vi "HFRR ADV v02.vi"() -> ()   [LabVIEW 2025] (continued)
            n2938 = property on="Sample Temperature ( °C )" class="XYGraph (strict)"("X Scale.Range:Minimum"=0.0, "X Scale.Range:Maximum"=75.0, "Y Scale.Range:Minimum"=58.0, "Y Scale.Range:Maximum"=62.0) -> ()  [unwired: 2 in, 2 out]
          }
        }
        n2939 = case shown="True" "RSTV1 3" {
          frame False {
          }
          frame True {
            n2940 = property on="Air Temperature  ( °C )" class="XYGraph (strict)"("Y Scale.Display Format:Precision"=u8 2 ("Y Scale.Format & Precision:Precision")) -> ()  [unwired: 2 in, 2 out]
            n2941 = property on="Air Temperature  ( °C )" class="XYGraph (strict)"("X Scale.Range:Minimum"=0.0 ("Y Scale.Range:Minimum"), "X Scale.Range:Maximum"=75.0 ("Y Scale.Range:Maximum"), "Y Scale.Range:Minimum"=20.0 ("X Scale.Range:Minimum"), "Y Scale.Range:Maximum"=26.0 ("X Scale.Range:Maximum")) -> ()  [unwired: 2 in, 2 out]
          }
        }
        n2942 = case shown="True" "RSTV1 4" {
          frame False {
          }
          frame True {
            n2943 = property on="Stroke ( mm )" class="XYGraph (strict)"("Y Scale.Display Format:Precision"=u8 2 ("Y Scale.Format & Precision:Precision")) -> ()  [unwired: 2 in, 2 out]
            n2944 = property on="Stroke ( mm )" class="XYGraph (strict)"("X Scale.Range:Minimum"=0.0 ("Y Scale.Range:Maximum"), "X Scale.Range:Maximum"=75.0 ("X Scale.Range:Minimum"), "Y Scale.Range:Minimum"=0.98, "Y Scale.Range:Maximum"=1.02) -> ()  [unwired: 2 in, 2 out]
          }
        }
        n2945 = case shown="True" "rstv2" {
          frame False {
          }
          frame True {
            n2946 = property on="Coefficient Of Friction" class="XYGraph (strict)"("Y Scale.Display Format:Precision"=u8 3 ("Y Scale.Format & Precision:Precision")) -> ()  [unwired: 2 in, 2 out]
            n2947 = property on="Coefficient Of Friction" class="XYGraph (strict)"("X Scale.Range:Minimum"=0.0 ("Y Scale.Range:Maximum"), "X Scale.Range:Maximum"=75.0, "Y Scale.Range:Minimum"=0.0, "Y Scale.Range:Maximum"=1.0 ("X Scale.Range:Minimum")) -> ()  [unwired: 2 in, 2 out]
          }
        }
        n2948 = case shown="True" "RST CP 3" {
          frame False {
          }
          frame True {
            n2949 = property on="Air Temp ( °C ) vs Humidity ( % RH )" class="XYGraph (strict)"("X Scale.Range:Minimum"=18.0, "X Scale.Range:Maximum"=28.0 ("X Scale.Range:Minimum"), "Y Scale.Range:Minimum"=30.0 ("X Scale.Range:Minimum"), "Y Scale.Range:Maximum"=70.0 ("X Scale.Range:Minimum")) -> ()  [unwired: 2 in, 2 out]
          }
        }
        n2950 = case shown="True" "OPEN 1" {
          frame False {
          }
          frame True {
            (unwired) 0  # existing file
            w3705 = "Choose a datalog file to open"  # prompt
            n2951 = local write "OPEN 1"(FALSE ("OPEN 1")) -> ()
            n2952 = String To Path(string="C:\\LAB-IQ\\Data\\") -> (path=w3690:path)
            n2953 = File Dialog(6:"*.dgf" ("pattern"), 7:w3705, 11:w3690) -> (0:w3688:errorcluster, 3:w3696:path)  [unwired: 4 in, 2 out]
            n2954 = Unbundle(w3688) -> ()  [unwired: 3 out]
            n2955 = Strip Path(path=w3696) -> (name=w3695:string)  [unwired: 1 out]
            n2956 = Path To String(path=w3696) -> (string=w3691:string)
            "string1" <- w3691
            n2957 = Match Pattern(string=w3695, regular expression=".dgf") -> (before substring=→"String Control":string)  [unwired: 1 in, 3 out]
            n2958 = Match Pattern(string=w3691, regular expression=".dgf" ("substring (\"\")")) -> (before substring=w3701:string)  [unwired: 1 in, 3 out]
            n2959 = Concatenate Strings(w3701, ".duf" ("Substring")) -> (w3697:string)
            n2960 = String To Path(string=w3697) -> (path=w3702:path)
            n2961 = call <vilib>:"Read Characters From File.vi"("file path (dialog if empty)"=w3702, "start of read offset (chars.:0)"=60 ("start of read offset (chars.: 0)")) -> ("character string"=→"String Control 2":string)  [unwired: 4 in, 3 out]
          }
        }
        n2962 = case shown="True" "OPEN 2" {
          frame False {
          }
          frame True {
            (unwired) 0  # existing file
            w3723 = "Choose a datalog file to open"  # prompt
            n2963 = local write "OPEN 2"(FALSE ("OPEN 1")) -> ()
            n2964 = String To Path(string="C:\\LAB-IQ\\Data\\") -> (path=w3708:path)
            n2965 = File Dialog(6:"*.dgf" ("pattern"), 7:w3723, 11:w3708) -> (0:w3706:errorcluster, 3:w3714:path)  [unwired: 4 in, 2 out]
            n2966 = Unbundle(w3706) -> ()  [unwired: 3 out]
            n2967 = Strip Path(path=w3714) -> (name=w3712:string)  [unwired: 1 out]
            n2968 = Path To String(path=w3714) -> (string=w3709:string)
            "string1 2" <- w3709
            n2969 = Match Pattern(string=w3712, regular expression=".dgf") -> (before substring=→"String Control 3":string)  [unwired: 1 in, 3 out]
            n2970 = Match Pattern(string=w3709, regular expression=".dgf" ("substring (\"\")")) -> (before substring=w3720:string)  [unwired: 1 in, 3 out]
            n2971 = Concatenate Strings(w3720, ".duf" ("Substring")) -> (w3717:string)
            n2972 = String To Path(string=w3717) -> (path=w3715:path)
            n2973 = call <vilib>:"Read Characters From File.vi"("file path (dialog if empty)"=w3715, "start of read offset (chars.:0)"=60 ("start of read offset (chars.: 0)")) -> ("character string"=→"String Control 4":string)  [unwired: 4 in, 3 out]
          }
        }
        n2974 = case shown="True" "OPEN 3" {
          frame False {
          }
          frame True {
            (unwired) 0  # existing file
            w3741 = "Choose a datalog file to open"  # prompt
            n2975 = local write "OPEN 3"(FALSE ("OPEN 1")) -> ()
            n2976 = String To Path(string="C:\\LAB-IQ\\Data\\") -> (path=w3726:path)
            n2977 = File Dialog(6:"*.dgf" ("pattern"), 7:w3741, 11:w3726) -> (0:w3724:errorcluster, 3:w3732:path)  [unwired: 4 in, 2 out]
            n2978 = Unbundle(w3724) -> ()  [unwired: 3 out]
            n2979 = Strip Path(path=w3732) -> (name=w3730:string)  [unwired: 1 out]
            n2980 = Path To String(path=w3732) -> (string=w3727:string)
            "string1 3" <- w3727
            n2981 = Match Pattern(string=w3730, regular expression=".dgf") -> (before substring=→"String Control 5":string)  [unwired: 1 in, 3 out]
            n2982 = Match Pattern(string=w3727, regular expression=".dgf" ("substring (\"\")")) -> (before substring=w3737:string)  [unwired: 1 in, 3 out]
            n2983 = Concatenate Strings(w3737, ".duf" ("Substring")) -> (w3734:string)
            n2984 = String To Path(string=w3734) -> (path=w3738:path)
            n2985 = call <vilib>:"Read Characters From File.vi"("file path (dialog if empty)"=w3738, "start of read offset (chars.:0)"=60 ("start of read offset (chars.: 0)")) -> ("character string"=→"String Control 6":string)  [unwired: 4 in, 3 out]
          }
        }
        n2986 = case shown="True" "OPEN 4" {
          frame False {
          }
          frame True {
            (unwired) 0  # existing file
            w3759 = "Choose a datalog file to open"  # prompt
            n2987 = local write "OPEN 4"(FALSE ("OPEN 1")) -> ()
            n2988 = String To Path(string="C:\\LAB-IQ\\Data\\") -> (path=w3744:path)
            n2989 = File Dialog(6:"*.dgf" ("pattern"), 7:w3759, 11:w3744) -> (0:w3742:errorcluster, 3:w3750:path)  [unwired: 4 in, 2 out]
            n2990 = Unbundle(w3742) -> ()  [unwired: 3 out]
            n2991 = Strip Path(path=w3750) -> (name=w3748:string)  [unwired: 1 out]
            n2992 = Path To String(path=w3750) -> (string=w3745:string)
            "string1 4" <- w3745
            n2993 = Match Pattern(string=w3748, regular expression=".dgf") -> (before substring=→"String Control 7":string)  [unwired: 1 in, 3 out]
            n2994 = Match Pattern(string=w3745, regular expression=".dgf" ("substring (\"\")")) -> (before substring=w3755:string)  [unwired: 1 in, 3 out]
            n2995 = Concatenate Strings(w3755, ".duf" ("Substring")) -> (w3752:string)
            n2996 = String To Path(string=w3752) -> (path=w3756:path)
            n2997 = call <vilib>:"Read Characters From File.vi"("file path (dialog if empty)"=w3756, "start of read offset (chars.:0)"=60 ("start of read offset (chars.: 0)")) -> ("character string"=→"String Control 8":string)  [unwired: 4 in, 3 out]
          }
        }
      }
      frame "About" {
        # "Elapsed time\ncof\nstroke\nmean pos\nTemp\nHumidity"
        n2998 = disable-structure shown="Disabled" {
          frame Disabled {
            n2999 = case shown="True" "Export" {
              frame False {
              }
              frame True {
                w3781 = "                                      " ("string")
                w3783 = "\r"
                (unwired) i16 6 ("width (-)")
                w3860 = "\r"
                w3792 = "\r"
                n3000 = local write "Export"(FALSE ("Export")) -> ()
                n3001 = local read "String 29"() -> (w3829:string)
                n3002 = local read "String 34"() -> (w3817:string)
                n3003 = local read "String 35"() -> (w3812:string)
                n3004 = local read "String 37"() -> (w3808:string)
                n3005 = local read "String 36"() -> (w3805:string)
                n3006 = local read "String 38"() -> (w3802:string)
                n3007 = local read "String 39"() -> (w3799:string)
                n3008 = Match Pattern(string=w3829, regular expression=".dwm") -> (before substring=w3825:string)  [unwired: 1 in, 3 out]
                "before substring" <- w3825
                n3009 = local read "S 38"() -> (w3820:string)
                n3010 = local read "S 39"() -> (w3813:string)
                n3011 = local read "Temperature before test 2"() -> (w3849:dbl)
                n3012 = local read "Temperature after test 2"() -> (w3854:dbl)
                n3013 = local read "Humidity before test 2"() -> (w3835:dbl)
                n3014 = local read "Humidity after test 2"() -> (w3850:dbl)
                n3015 = local read "MWSD 2"() -> (w3846:dbl)
                n3016 = local read "WS1.4 2"() -> (w3862:dbl)
                n3017 = local read "HCF 2"() -> (w3858:dbl)
                n3018 = local read "AVP 2"() -> (w3847:dbl)
                n3019 = Concatenate Strings("1," ("string"), w3820) -> (w3819:string)
                n3020 = Concatenate Strings("2," ("string"), w3817) -> (w3816:string)
                n3021 = Concatenate Strings("3," ("string"), w3813) -> (w3815:string)
                n3022 = Concatenate Strings("4," ("string"), w3812) -> (w3811:string)
                n3023 = Concatenate Strings("5," ("string"), w3808) -> (w3809:string)
                n3024 = Concatenate Strings("6," ("string"), w3805) -> (w3806:string)
                n3025 = Concatenate Strings("7," ("string"), w3802) -> (w3803:string)
                n3026 = Concatenate Strings("8," ("string"), w3799) -> (w3800:string)
                n3027 = local read "Sample ID"() -> (w3867:string)
                n3028 = case shown="\"xlx\"" "Select File Type" {
                  tunnel: w3825 -> [w3870 w3872 w3874]
                  tunnel: [w3868 w3873 w3875] -> w3824
                  frame "xlx" {
                    n3029 = Concatenate Strings(w3870, ".xls" ("string")) -> (w3868:string)
                  }
                  frame "csv" {
                    n3030 = Concatenate Strings(w3872, ".csv" ("string")) -> (w3873:string)
                  }
                  frame "txt" {
                    n3031 = Concatenate Strings(w3874, ".txt" ("string")) -> (w3875:string)
                  }
                }
                n3032 = local read "Test Date"() -> (w3866:string)
                n3033 = local read "String 45"() -> (w3780:string)
                n3034 = local read "String 31"() -> (w3865:string)
                n3035 = local read "String 32"() -> (w3864:string)
                n3036 = local read "TITTLE"() -> (w3788:string)
                n3037 = Number To Fractional String(number=w3835, width (-)=i16 6, precision (6)=i16 2) -> (F-format string=w3834:string)  [unwired: 1 in]
                n3038 = Number To Fractional String(number=w3849, width (-)=i16 6, precision (6)=i16 2) -> (F-format string=w3855:string)  [unwired: 1 in]
                n3039 = Number To Fractional String(number=w3850, width (-)=i16 6, precision (6)=i16 2) -> (F-format string=w3848:string)  [unwired: 1 in]
                n3040 = Number To Fractional String(number=w3854, width (-)=i16 6, precision (6)=i16 2) -> (F-format string=w3853:string)  [unwired: 1 in]
                n3041 = Number To Fractional String(number=w3846, width (-)=i16 6, precision (6)=i16 2) -> (F-format string=w3844:string)  [unwired: 1 in]
                n3042 = Number To Fractional String(number=w3847, width (-)=i16 6, precision (6)=i16 2) -> (F-format string=w3845:string)  [unwired: 1 in]
                n3043 = Number To Fractional String(number=w3858, width (-)=i16 6, precision (6)=i16 2) -> (F-format string=w3859:string)  [unwired: 1 in]
                n3044 = Number To Fractional String(number=w3862, precision (6)=i16 2) -> (F-format string=w3863:string)  [unwired: 2 in]
                n3045 = local read "s.NO"() -> (w3782:string)
                n3046 = Concatenate Strings("=" ("string"), w3788) -> (w3787:string)
                n3047 = Concatenate Strings("S.No," ("string"), "                                       Parameters" ("string")) -> (w3793:string)
                n3048 = Concatenate Strings(w3860, w3819, w3834, w3860, w3816, w3855, w3860, w3815, w3848, w3860, w3811, w3853, w3860, w3809, w3844, w3860, w3806, w3845, w3860, w3803, w3859, w3860, w3800, w3863) -> (w3822:string)
                n3049 = Concatenate Strings(w3792, "," ("string"), w3780, w3782, w3781, w3864, w3867, w3781, w3865, w3866, w3792) -> (w3790:string)
                n3050 = local read "Tested by"() -> (w3796:string)
                n3051 = local read "String 33"() -> (w3797:string)
                n3052 = Concatenate Strings("," ("string"), "                                                                             " ("string")) -> (w3785:string)
                n3053 = Concatenate Strings(w3787, w3783, w3790, w3783, w3793, w3822, w3783, w3785, w3797, w3796) -> (→"export":string)
                n3054 = String To Path(string=w3824) -> (path=w3831:path)
                n3055 = local read "export"() -> (w3826:string)
                n3056 = call <vilib>:"Write Characters To File.vi"("append to file? (new file:F)"=FALSE, "character string"=w3826, "file path (dialog if empty)"=w3831) -> ()  [unwired: 2 in, 1 out]
              }
            }
          }
          frame Enabled {
          }
        }
        n3057 = case shown="True" "OK Button 17" {
          frame False {
          }
          frame True {
            (unwired) 0  # existing file
            w4084 = "Choose a datalog file to open"  # prompt
            n3058 = local write "OK Button 17"(FALSE ("OK Button 17")) -> ()
            n3059 = local read "String"() -> (w4079:string)
            n3060 = String To Path(string=w4079) -> (path=w4080:path)
            n3061 = File Dialog(6:"*.duf" ("pattern"), 7:w4084, 11:w4080) -> (0:w4071:errorcluster, 3:w4090:path)  [unwired: 4 in, 2 out]
            n3062 = Unbundle(w4071) -> ()  [unwired: 3 out]
            n3063 = Open/Create/Replace File "Open File"(file path (use dialog)=w4090) -> (refnum out=w4082:refnum<file>)  [unwired: 5 in, 2 out]
            n3064 = Strip Path(path=w4090) -> (name=w4088:string)  [unwired: 1 out]
            n3065 = Path To String(path=w4090) -> (string=w4073:string)
            n3066 = while {
              tunnel: w4082 -> [w4094]
              i -> [w4091]
              stop <- w4092 continue-if-true
              (unwired) TRUE ("line mode (F)")
              n3067 = Read from Text File "Read File"(file (use dialog)=w4094) -> (text=w4093:string)  [unwired: 3 in, 3 out]
              n3068 = local write "Numeric 16"(w4091) -> ()
              n3069 = String Length(string=w4093) -> (length=w4096:i32)
              n3070 = Greater?(x=w4096, y=1) -> (0:w4092:bool)
            }
            n3071 = local write "String 29"(w4073) -> ()
            n3072 = Search and Replace String(input string=w4073, search string=".duf", replace string=".dgf" ("replace string (\"\")")) -> (result string=→"String Indicator 4":string)  [unwired: 5 in, 3 out]
            n3073 = Match Pattern(string=w4088, regular expression=".dwm") -> (before substring=w4072:string)  [unwired: 1 in, 3 out]
            "String Indicator" <- w4072
            n3074 = Match Pattern(string=w4073, regular expression=".dwm" ("substring (\"\")")) -> (before substring=w4074:string)  [unwired: 1 in, 3 out]
            "String Indicator 3" <- w4074
            n3075 = local write "TITTLE 2"(w4072) -> ()
            n3076 = String To Path(string=w4074) -> (path=w4081:path)
            "path" <- w4081
            n3077 = call <vilib>:"Read Characters From File.vi"("file path (dialog if empty)"=w4081, "start of read offset (chars.:0)"=60 ("start of read offset (chars.: 0)")) -> ("character string"=→"String Indicator 2":string)  [unwired: 4 in, 3 out]
          }
        }
        n3078 = call <vilib>:"Query Available Printers.vi"() -> ("system configured printers"=w3773:string[])  [unwired: 9 in, 2 out]
        "System Configured Printers 2" <- w3773
        n3079 = local read "OK Button 16"() -> (w3770:bool)
        n3080 = case shown="True" "OK Button 16" {
          frame False {
          }
          frame True {
            n3081 = stacked-sequence {
              frame #0 {
                n3082 = local read "Numeric 16"() -> (w4098:i32)
                n3083 = local write "Numeric 10"(w4098) -> ()
              }
              frame #1 {
                n3084 = local read "String 29"() -> (w4101:string)
                n3085 = String To Path(string=w4101) -> (path=w4100:path)
                n3086 = Open/Create/Replace File "Open File"(file path (use dialog)=w4100) -> (refnum out=w4102:refnum<file>)  [unwired: 5 in, 2 out]
                n3087 = for {
                  N: 16 -> [_]
                  tunnel: w4102 -> [w4109]
                  i -> [w4105]
                  (unwired) TRUE ("line mode (F)")
                  n3088 = Read from Text File "Read File"(file (use dialog)=w4109) -> (text=w4103:string)  [unwired: 3 in, 3 out]
                  n3089 = Match Pattern(string=w4103, regular expression="(") -> (after substring=w4108:string)  [unwired: 1 in, 3 out]
                  n3090 = Match Pattern(string=w4108, regular expression=")") -> (before substring=w4104:string)  [unwired: 1 in, 3 out]
                  n3091 = case shown="1" w4105 {
                    tunnel: w4104 -> [w4110 w4111 _ _ w4112 w4113 w4114 w4116 w4118 w4120 w4122 w4124 w4126 w4128 _]
                    tunnel: w4103 -> [_ _ _ _ _ _ _ _ _ _ _ _ _ _ _]
                    frame 0 {
                      "TITTLE" <- w4110
                    }
                    frame 1 {
                      "Sample ID" <- w4111
                    }
                    frame 2 {
                    }
                    frame 3 {
                    }
                    frame 4 {
                      "Test Date" <- w4112
                    }
                    frame 5 {
                      "Tested by" <- w4113
                    }
                    frame 6 {
                      n3092 = Fract/Exp String To Number(string=w4114) -> (number=→"Humidity before test 2":dbl)  [unwired: 3 in, 1 out]
                    }
                    frame 7 {
                      n3093 = Fract/Exp String To Number(string=w4116) -> (number=→"Temperature before test 2":dbl)  [unwired: 3 in, 1 out]
                    }
                    frame 8 {
                      n3094 = Fract/Exp String To Number(string=w4118) -> (number=→"Humidity after test 2":dbl)  [unwired: 3 in, 1 out]
                    }
                    frame 9 {
                      n3095 = Fract/Exp String To Number(string=w4120) -> (number=→"Temperature after test 2":dbl)  [unwired: 3 in, 1 out]
                    }
                    frame 10 {
                      n3096 = Fract/Exp String To Number(string=w4122) -> (number=→"MWSD 2":dbl)  [unwired: 3 in, 1 out]
                    }
                    frame 11 {
                      n3097 = Fract/Exp String To Number(string=w4124) -> (number=→"AVP 2":dbl)  [unwired: 3 in, 1 out]
                    }
                    frame 12 {
                      n3098 = Fract/Exp String To Number(string=w4126) -> (number=→"HCF 2":dbl)  [unwired: 3 in, 1 out]
                    }
                    frame 13 {
                      n3099 = Fract/Exp String To Number(string=w4128) -> (number=→"WS1.4 2":dbl)  [unwired: 3 in, 1 out]
                    }
                    frame 14, Default {
                    }
                  }
                }
              }
              frame #2 {
              }
            }
            n3100 = local write "OK Button 16"(FALSE ("OK Button 13")) -> ()
          }
        }
        n3101 = Index Array(array=w3773, index="Select Printer 3") -> (element=w3775:string)
        "Selected Printer" <- w3775
        n3102 = case shown="True" w3770 {
          frame False {
          }
          frame True {
            n3103 = flat-sequence {
              frame #0 {
              }
              frame #1 {
                n3104 = Wait (ms)(milliseconds to wait=u32 100) -> ()  [unwired: 1 out]
              }
              frame #2 {
                n3105 = local write "OK Button 16"(FALSE ("Print 3")) -> ()
              }
            }
          }
        }
        n3106 = case shown="True" "Print" {
          tunnel: w3775 -> [_ w4067]
          frame False {
          }
          frame True {
            (unwired) i16 6 ("width (-)")
            (unwired) "TESTED BY : "
            (unwired) "TESTED DATE :"
            (unwired) "SAMPLE ID : "
            (unwired) "SAMPLE DESIGN : "
            w4025 = "\r"
            w4042 = "\r"
            # "add image"
            n3107 = local read "Sample ID"() -> (w4015:string)
            n3108 = local read "Tested by"() -> (w4018:string)
            n3109 = local read "String 34"() -> (w4005:string)
            n3110 = local read "String 45"() -> (w3985:string)
            n3111 = local read "String 35"() -> (w4000:string)
            n3112 = local read "String 37"() -> (w3998:string)
            n3113 = local read "String 32"() -> (w4020:string)
            n3114 = local read "String 36"() -> (w3995:string)
            n3115 = local read "String 31"() -> (w4019:string)
            n3116 = local read "Test Date"() -> (w4016:string)
            n3117 = local read "String 33"() -> (w4021:string)
            n3118 = local read "String 38"() -> (w3991:string)
            n3119 = local read "String 39"() -> (w3988:string)
            n3120 = local write "Print"(FALSE ("Print FF")) -> ()
            n3121 = local read "S 39"() -> (w4003:string)
            n3122 = local read "S 38"() -> (w4010:string)
            n3123 = local read "Temperature before test 2"() -> (w4041:dbl)
            n3124 = local read "Temperature after test 2"() -> (w4031:dbl)
            n3125 = local read "Humidity before test 2"() -> (w4056:dbl)
            n3126 = local read "Humidity after test 2"() -> (w4040:dbl)
            n3127 = local read "MWSD 2"() -> (w4045:dbl)
            n3128 = local read "WS1.4 2"() -> (w4023:dbl)
            n3129 = Concatenate Strings("2)" ("string"), w4005) -> (w4006:string)
            n3130 = Concatenate Strings("3)" ("string"), w4003) -> (w4004:string)
            n3131 = Concatenate Strings("1)" ("string"), w4010) -> (w4009:string)
            n3132 = Concatenate Strings("4)" ("string"), w4000) -> (w4001:string)
            n3133 = Concatenate Strings("5)" ("string"), w3998) -> (w3997:string)
            n3134 = Concatenate Strings("6)" ("string"), w3995) -> (w3994:string)
            n3135 = Concatenate Strings("7)" ("string"), w3991) -> (w3992:string)
            n3136 = Concatenate Strings("8)" ("string"), w3988) -> (w3989:string)
            n3137 = local read "HCF 2"() -> (w4027:dbl)
            n3138 = local read "AVP 2"() -> (w4044:dbl)
            n3139 = local read "s.NO"() -> (w3986:string)
            n3140 = call <vilib>:"New Report.vi"("report type"=enum16{"Standard Report", "HTML"}."Standard Report") -> ("report out"=w4065:refnum<class "NI_report.lvclass">, "error out"=w4064:errorcluster)  [unwired: 13 in]
            n3141 = local read "TITTLE"() -> (w4017:string)
            n3142 = Concatenate Strings(w4042, w3985, w3986, w4042, w4020, w4015, w4042, w4019, w4016, w4042, w4021, w4018, w4042) -> (w4035:string)
            "test by" <- w4035
            n3143 = Number To Fractional String(number=w4041, width (-)=i16 6, precision (6)=i16 2) -> (F-format string=w4030:string)  [unwired: 1 in]
            n3144 = Number To Fractional String(number=w4040, width (-)=i16 6, precision (6)=i16 2) -> (F-format string=w4043:string)  [unwired: 1 in]
            n3145 = Number To Fractional String(number=w4056, width (-)=i16 6, precision (6)=i16 2) -> (F-format string=w4061:string)  [unwired: 1 in]
            n3146 = Number To Fractional String(number=w4045, width (-)=i16 6, precision (6)=i16 2) -> (F-format string=w4047:string)  [unwired: 1 in]
            n3147 = Number To Fractional String(number=w4031, width (-)=i16 6, precision (6)=i16 2) -> (F-format string=w4032:string)  [unwired: 1 in]
            n3148 = Number To Fractional String(number=w4044, width (-)=i16 6, precision (6)=i16 2) -> (F-format string=w4046:string)  [unwired: 1 in]
            n3149 = Number To Fractional String(number=w4027, width (-)=i16 6, precision (6)=i16 2) -> (F-format string=w4026:string)  [unwired: 1 in]
            n3150 = Number To Fractional String(number=w4023, precision (6)=i16 2) -> (F-format string=w4022:string)  [unwired: 2 in]
            n3151 = call-dynamic "Set Report Header Text.vi"("report in"=w4065, "center header text"=w4017, "error in (no error)"=w4064) -> ("report out"=w4036:refnum<class "NI_report.lvclass">, "error out"=w4037:errorcluster)  [unwired: 11 in]
            n3152 = Concatenate Strings(w4025, w4009, w4061, w4025, w4006, w4030, w4025, w4004, w4043, w4025, w4001, w4032, w4025, w3997, w4047, w4025, w3994, w4046, w4025, w3992, w4026, w4025, w3989, w4022) -> (w4013:string)
            "export 2" <- w4013
            n3153 = call-poly <vilib>:"Append Report Text.vi"("report in"=w4036, "text"=w4035, "error in (no error)"=w4037) -> ("report out"=w4039:refnum<class "NI_report.lvclass">, "error out"=w4038:errorcluster)  [unwired: 9 in, 2 out]
            n3154 = local read "test by"() -> (w4012:string)
            n3155 = local read "TITTLE"() -> (w4014:string)
            n3156 = call-poly <vilib>:"Append Report Text.vi"("report in"=w4039, "error in (no error)"=w4038) -> ("report out"=w4060:refnum<class "NI_report.lvclass">, "error out"=w4058:errorcluster)  [unwired: 10 in, 2 out]
            n3157 = Concatenate Strings(w4014, w4013, w4012) -> (→"output":string)
            n3158 = call-poly <vilib>:"Append Report Text.vi"("report in"=w4060, "text"=w4013, "error in (no error)"=w4058) -> ("report out"=w4059:refnum<class "NI_report.lvclass">, "error out"=w4057:errorcluster)  [unwired: 9 in, 2 out]
            n3159 = call-dynamic "Print Report.vi"("report in"=w4059, "printer name (default)"=w4067, "error in (no error)"=w4057) -> ("report out"=w4069:refnum<class "NI_report.lvclass">, "error out"=w4070:errorcluster)  [unwired: 11 in]
            n3160 = call-dynamic "Dispose Report.vi"("report in"=w4069, "error in (no error)"=w4070) -> ()  [unwired: 13 in, 1 out]
          }
        }
        n3161 = case shown="True" "Print 2" {
          frame False {
          }
          frame True {
            n3162 = flat-sequence {
              frame #0 {
                n3163 = local read "s.NO"() -> (→"s.NO 2":string)
                n3164 = Wait (ms)(milliseconds to wait=u32 20) -> ()  [unwired: 1 out]
                n3165 = local read "Sample ID  3"() -> (→"Sample ID  6":string)
                n3166 = local read "Sample ID  4"() -> (→"Sample ID  7":string)
                n3167 = local read "Sample ID"() -> (→"Sample ID  2":string)
                n3168 = local read "Tested by"() -> (→"Tested by 2":string)
                n3169 = local read "Test Date"() -> (→"Test Date 2":string)
                n3170 = local read "Humidity after test 3"() -> (→"Humidity after test 4":dbl)
                n3171 = local read "Ref A Test Date :"() -> (→"TITTLE 4":string)
                n3172 = local read "Temperature before test 3"() -> (w3892:dbl)
                n3173 = local read "Temperature before test 3"() -> (→"Temperature after test 5":dbl)
                n3174 = local read "Temperature after test 3"() -> (→"Temperature after test 4":dbl)
                n3175 = local read "Humidity before test 3"() -> (→"Humidity before test 4":dbl)
                n3176 = local write "Temperature before test 3"(w3892) -> ()
                n3177 = local read "image data"() -> (w3883:T2)
                n3178 = String To Path(string="C:\\LAB-IQ\\im\\Temp_resized.jpg") -> (path=w3884:path)
                "path 2" <- w3884
                n3179 = call <vilib>:"Write JPEG File.vi"("image data"=w3883, "path to JPEG file"=w3884) -> ()  [unwired: 8 in, 2 out]
                "Ref A Test Date :" <- "Ref A Test Date :"
                "Ref B Test Date :" <- "Ref B Test Date :"
                "Ref B Scar Value :" <- "Ref B Scar Value :"
                "Ref A Scar Value :" <- "Ref A Scar Value :"
              }
              frame #1 {
                (unwired) HTML_Report_Image_Alignment."MIDDLE" ("alignment (default)")
                w3920 = u16 0 items=["portrait", "landscape"] ("orientation (portrait)")
                (unwired) HTML_Report_Image_Alignment."ABSMIDDLE" ("alignment (default)")
                (unwired) "TESTED BY : "
                (unwired) "TESTED DATE :"
                (unwired) "SAMPLE ID : "
                (unwired) "SAMPLE DESIGN : "
                w3953 = "\r"
                # "add image"
                n3180 = Wait (ms)(milliseconds to wait=u32 20) -> ()  [unwired: 1 out]
                n3181 = local read "Sample ID  2"() -> (w3946:string)
                n3182 = local read "Wear Scar X"() -> (w3918:dbl)
                "Length ( microns ) 2" <- w3918
                n3183 = local read "Wear Scar Y"() -> (w3917:dbl)
                "Wear Scar Y ( microns ) :" <- w3917
                n3184 = local read "Test Date 2"() -> (w3947:string)
                n3185 = local read "Tested by 2"() -> (w3948:string)
                n3186 = local read "String 46"() -> (w3944:string)
                n3187 = local read "String 48"() -> (w3950:string)
                n3188 = local read "String 47"() -> (w3949:string)
                n3189 = local read "String 49"() -> (w3951:string)
                n3190 = local read "String 10"() -> (w3904:string)
                n3191 = local read "s.NO 2"() -> (w3945:string)
                n3192 = Add(x=w3918, y=w3917) -> (x+y=w3916:dbl)
                n3193 = call <vilib>:"New Report.vi"("report type"=enum16{"Standard Report", "HTML"}."HTML") -> ("report out"=w3924:refnum<class "NI_report.lvclass">, "error out"=w3922:errorcluster)  [unwired: 13 in]
                n3194 = Concatenate Strings(w3953, w3944, w3945, w3953, w3950, w3946, w3953, w3949, w3947, w3953, w3951, w3948, w3953) -> (→"test by 2":string)
                n3195 = Concatenate Strings("C:\\LAB-IQ\\Data\\" ("string"), w3904, ".jpg" ("string")) -> ()  [unwired: 1 out]
                n3196 = Divide(x=w3916, y=2.0) -> (x/y=→"Mean Wear ( microns) :":dbl)
                n3197 = call-dynamic "Set Report Orientation.vi"("report in"=w3924, "orientation (portrait)"=w3920, "error in (no error)"=w3922) -> ("report out"=w3923:refnum<class "NI_report.lvclass">, "error out"=w3921:errorcluster)  [unwired: 11 in]
                n3198 = for {
                  N: 5 -> [_]
                  tunnel: w3923 -> [w3974]
                  tunnel: [w3973] -> w3902
                  tunnel: w3921 -> [w3972]
                  tunnel: [w3971] -> w3901
                  n3199 = call-dynamic "Set Report Tab Width.vi"("report in"=w3974, "error in (no error)"=w3972) -> ("report out"=w3973:refnum<class "NI_report.lvclass">, "error out"=w3971:errorcluster)  [unwired: 12 in]
                }
                n3200 = local read "TITTLE"() -> (w3919:string)
                n3201 = call-dynamic "Set Report Header Text.vi"("report in"=w3902, "center header text"=w3919, "error in (no error)"=w3901) -> ("report out"=w3940:refnum<class "NI_report.lvclass">, "error out"=w3939:errorcluster)  [unwired: 11 in]
                n3202 = for {
                  N: 1 -> [_]
                  tunnel: [w3978] -> w3926
                  tunnel: [w3977] -> w3925
                  tunnel: w3940 -> [w3976]
                  tunnel: w3939 -> [w3975]
                  n3203 = call-dynamic "New Report Line.vi"("report in"=w3976, "error in (no error)"=w3975) -> ("report out"=w3978:refnum<class "NI_report.lvclass">, "error out"=w3977:errorcluster)  [unwired: 12 in]
                }
                n3204 = for {
                  N: 2 -> [_]
                  tunnel: [w3970] -> w3932
                  tunnel: [w3969] -> w3931
                  tunnel: w3926 -> [w3968]
                  tunnel: w3925 -> [w3967]
                  n3205 = call-dynamic "New Report Line.vi"("report in"=w3968, "error in (no error)"=w3967) -> ("report out"=w3970:refnum<class "NI_report.lvclass">, "error out"=w3969:errorcluster)  [unwired: 12 in]
                }
                n3206 = for {
                  N: 25 -> [_]
                  tunnel: w3932 -> [w3966]
                  tunnel: w3931 -> [w3964]
                  tunnel: [w3965] -> w3935
                  tunnel: [w3963] -> w3934
                  n3207 = call-dynamic "Set Report Tab Width.vi"("report in"=w3966, "error in (no error)"=w3964) -> ("report out"=w3965:refnum<class "NI_report.lvclass">, "error out"=w3963:errorcluster)  [unwired: 12 in]
                }
                n3208 = control-ref of="Tab Control 9"() -> (w3930:refnum<vi>)
                n3209 = call-dynamic "Append Control Image to Report.vi"("report in"=w3935, "alignment (default)"=HTML_Report_Image_Alignment."ABSMIDDLE", "ctrl reference"=w3930, "error in (no error)"=w3934) -> ("report out"=w3929:refnum<class "NI_report.lvclass">, "error out"=w3928:errorcluster)  [unwired: 8 in, 2 out]
                n3210 = for {
                  N: 3 -> [_]
                  tunnel: [w3962] -> w3913
                  tunnel: [w3961] -> w3912
                  tunnel: w3929 -> [w3960]
                  tunnel: w3928 -> [w3959]
                  n3211 = call-dynamic "New Report Line.vi"("report in"=w3960, "error in (no error)"=w3959) -> ("report out"=w3962:refnum<class "NI_report.lvclass">, "error out"=w3961:errorcluster)  [unwired: 12 in]
                }
                n3212 = for {
                  N: 100 -> [_]
                  tunnel: w3913 -> [w3958]
                  tunnel: w3912 -> [w3956]
                  tunnel: [w3957] -> w3909
                  tunnel: [w3955] -> w3907
                  n3213 = call-dynamic "Set Report Tab Width.vi"("report in"=w3958, "error in (no error)"=w3956) -> ("report out"=w3957:refnum<class "NI_report.lvclass">, "error out"=w3955:errorcluster)  [unwired: 12 in]
                }
                n3214 = String To Path(string="C:\\LAB-IQ\\im\\Temp_resized.jpg") -> (path=w3899:path)
                n3215 = call-poly <vilib>:"Append Image to Report.vi"("report in"=w3909, "path or URL of image"=w3899, "error in (no error)"=w3907) -> ("report out"=w3908:refnum<class "NI_report.lvclass">, "error out"=w3906:errorcluster)  [unwired: 9 in, 2 out]
                n3216 = call-poly <vilib>:"Open HTML Report in Browser.vi"("report in"=w3908, "error in (no error)"=w3906) -> ("report out"=w3943:refnum<class "NI_report.lvclass">, "error out"=w3942:errorcluster)  [unwired: 11 in, 1 out]
                n3217 = call-dynamic "Dispose Report.vi"("report in"=w3943, "error in (no error)"=w3942) -> ()  [unwired: 13 in, 1 out]
              }
              frame #2 {
              }
              frame #3 {
                n3218 = disable-structure shown="Disabled" {
                  frame Disabled {
                    n3219 = local read "String 10"() -> (w3983:string)
                    n3220 = Concatenate Strings("C:\\LAB-IQ-NXT\\Data\\" ("string"), w3983, ".jpg" ("string")) -> (w3981:string)
                    n3221 = String To Path(string=w3981) -> (path=w3980:path)
                    n3222 = Delete(path (use dialog)=w3980) -> ()  [unwired: 4 in, 3 out]
                  }
                  frame Enabled {
                  }
                }
                n3223 = local write "Print 2"(FALSE ("Print")) -> ()
              }
            }
          }
        }
      }
    }
    n3224 = Wait (ms)(milliseconds to wait=u32 50) -> ()  [unwired: 1 out]
    n3225 = Wait (ms)(milliseconds to wait=u32 50) -> ()  [unwired: 1 out]
    n3226 = local read "Quit"() -> (w2344:bool)
  }
  n3227 = VISA Close(VISA resource name=w46, error in (no error)=w45) -> ()  [unwired: 1 out]
  n3228 = while {
    stop <- w4134 stop-if-true
    # "DEMO"
    n3229 = local read "Auto Start Test"() -> (w4132:bool)
    n3230 = Wait (ms)(milliseconds to wait=u32 1000) -> ()  [unwired: 1 out]
    n3231 = local read "RUN"() -> (w4131:bool)
    n3232 = Or(x=w4131, y=w4132) -> (x .or. y?=w4130:bool)
    n3233 = case shown="True" w4130 {
      frame False {
      }
      frame True {
        n3234 = local read "LVDT STROKE Actual"() -> (w4136:dbl)
        n3235 = local read "DEMO MODE"() -> (w4135:bool)
        n3236 = case shown="True" w4135 {
          frame False {
          }
          frame True {
            n3237 = call-poly <vilib>:"Random Number (Range).vi"("lower bound (0)"=22.0 ("upper bound (100)"), "upper bound (100)"=24.0) -> ("number"=w4144:dbl)  [unwired: 9 in]
            n3238 = local write "AIR TEMP"(w4144) -> ()
          }
        }
        n3239 = In Range and Coerce(upper limit=1.2, x=w4136, lower limit=0.6) -> (In Range?=w4139:bool)  [unwired: 1 out]
        n3240 = call-poly <vilib>:"Random Number (Range).vi"("lower bound (0)"=0.998 ("upper bound (100)"), "upper bound (100)"=1.003) -> ("number"=w4137:dbl)  [unwired: 9 in]
        n3241 = case shown="True" w4139 {
          tunnel: [w4147 w4148] -> w4138
          tunnel: w4137 -> [_ w4148]
          tunnel: w4136 -> [w4147 _]
          frame False {
          }
          frame True {
          }
        }
        "LVDT STROKE DISPLAY" <- w4138
      }
    }
    n3242 = local read "Quit"() -> (w4134:bool)
  }
  n3243 = while {
    tunnel: [w4165] -> w52
    shift-right: [w4158] -> _
    shift-left: 0.0 -> [w4161]
    shift-right: [w4157] -> _
    shift-left: 0.0 -> [w4160]
    shift-right: [w4156] -> _
    shift-left: 100.0 ("vc_cmd") -> [w4159]
    stop <- w4165 stop-if-true
    # "PID LOGIC"
    n3244 = local read "run test Calibration"() -> (w4153:bool)
    n3245 = local read "RUN"() -> (w4163:bool)
    n3246 = local read "Auto Start Temp"() -> (w4154:bool)
    n3247 = local read "Auto Start Test"() -> (w4162:bool)
    n3248 = local read "START TEMP"() -> (w4152:bool)
    n3249 = And(x=w4154, y=w4162) -> (x .and. y?=w4155:bool)
    n3250 = Or(x=w4163, y=w4155) -> (x .or. y?=w4164:bool)
    n3251 = And(x=w4164, y=w4152) -> (x .and. y?=w4151:bool)
    n3252 = And(x=w4153, y=w4152) -> (x .and. y?=w4150:bool)
    n3253 = Or(x=w4150, y=w4151) -> (x .or. y?=w4149:bool)
    n3254 = Wait (ms)(milliseconds to wait="milliseconds to wait") -> ()  [unwired: 1 out]
    n3255 = case shown="True" w4149 {
      tunnel: [400.0 ("out_vc_cmd") w4184] -> w4156
      tunnel: [w4168 w4186] -> w4157
      tunnel: [w4168 w4185] -> w4158
      tunnel: w4161 -> [_ w4175]
      tunnel: w4160 -> [_ w4174]
      tunnel: w4159 -> [_ w4173]
      tunnel: w4153 -> [_ w4169]
      frame False {
        w4168 = 0.0 ("error_out")
      }
      frame True {
        n3256 = case shown="True" w4169 {
          tunnel: [w4193 1.0] -> w4171
          frame False {
            n3257 = local read "Set Strk"() -> (w4192:dbl)
            n3258 = Add(x=w4192, y="Add up Stroke") -> (x+y=w4193:dbl)
          }
          frame True {
          }
        }
        n3259 = local read "LVDT STROKE"() -> (w4170:dbl)
        n3260 = formula code="// Zero-Hardcode Explicit Positional-Form PID Engine\n// Inputs: target_stroke, measured_stroke, dt, prev_error, integral_accumulator_in, prev_vc_cmd\n//         kp, ki, kd, max_step_change, max_amplitude, min_amplitude, startup_cmd\n// Outputs: vc_cmd, error_out, out_error, integral_accumulator_out, out_vc_cmd\n\n// 1. Calculate Tracking Error\nfloat current_error = target_stroke - measured_stroke;\nerror_out = current_error;\n\n// 2. Compute Proportional Term\nfloat p_term = kp * current_error;\n\n// 3. Compute Derivative Term\nfloat d_term = 0.0;\nif (dt > 0.0) {\n    d_term = kd * ((current_error - prev_error) / dt);\n}\n\n// 4. Update and Accumulate Integral Term\nfloat current_integral = integral_accumulator_in + (current_error * dt);\nfloat i_term = ki * current_integral;\n\n// 5. Calculate Ideal Target Command (Anchored by startup baseline)\nfloat ideal_command = startup_cmd + p_term + i_term + d_term;\n\n// 6. Apply Loop Rate Limiting FIRST \n// (Forces the command to climb gradually from prev_vc_cmd instead of jumping straight to max)\nfloat raw_adjustment = ideal_command - prev_vc_cmd;\n\nif (raw_adjustment > max_step_change) {\n    raw_adjustment = max_step_change;\n} else if (raw_adjustment < -max_step_change) {\n    raw_adjustment = -max_step_change;\n}\n\nfloat next_vc_cmd = prev_vc_cmd + raw_adjustment;\n\n// 7. Anti-Windup Protection & Final Output Safety Safeguard Clamping\n// (Back-calculating based on what we are ACTUALLY outputting)\nif (next_vc_cmd > max_amplitude) {\n    float excess = next_vc_cmd - max_amplitude;\n    if (ki > 0.0) {\n        current_integral -= excess / ki;\n    }\n    next_vc_cmd = max_amplitude;\n} else if (next_vc_cmd < min_amplitude) {\n    float excess = next_vc_cmd - min_amplitude;\n    if (ki > 0.0) {\n        current_integral -= excess / ki;\n    }\n    next_vc_cmd = min_amplitude;\n}\n\n// 8. Map to Shift Registers for memory persistence\nvc_cmd = next_vc_cmd;\nout_error = current_error;                   \nintegral_accumulator_out = current_integral;  \nout_vc_cmd = next_vc_cmd;"("target_stroke"=w4171, "measured_stroke"=w4170, "dt"="dt", "integral_accumulator_in"=w4174, "prev_error"=w4175, "prev_vc_cmd"=w4173, "kp"="kp", "ki"="ki", "kd"="kd", "max_step_change"="max_step_change", "max_amplitude"="max_amplitude", "min_amplitude"="min_amplitude", "startup_cmd"="startup_cmd") -> ("vc_cmd"=w4190:dbl, "out_error"=w4185:dbl, "integral_accumulator_out"=w4186:dbl, "out_vc_cmd"=w4184:dbl)  [unwired: 1 out]
        "output Vpp" <- w4190
        n3261 = Number To Fractional String(number=w4190, precision (6)=i16 1) -> (F-format string=w4188:string)  [unwired: 2 in]
        n3262 = Concatenate Strings("DAC;" ("string"), w4188) -> (w4172:string)
        n3263 = local write "Due Write"(w4172) -> ()
        "prev_error" <- w4175
        "integral_accumulator_in" <- w4174
        "prev_vc_cmd" <- w4173
      }
    }
    n3264 = local read "Quit"() -> (w4165:bool)
  }
  n3265 = Or(x=w47, y=w49) -> (x .or. y?=w54:bool)
  n3266 = control-ref of="new picture"() -> ()  [unwired: 1 out]
  n3267 = Or(x=w57, y=w54) -> (x .or. y?=w51:bool)
  n3268 = Or(x=w51, y=w52) -> (x .or. y?=w48:bool)
  n3269 = while {
    tunnel: [w4195] -> w56
    i -> [w4202]
    stop <- w4195 stop-if-true
    n3270 = local read "Quit"() -> (w4195:bool)
    n3271 = Equal To 0?(x=w4202) -> (x = 0?=w4200:bool)
    n3272 = call "Elapsed Time3"("Time Target (s)"=45.0, "Auto Reset"=TRUE) -> ("Time has Elapsed"=w4199:bool)  [unwired: 10 in, 7 out]
    n3273 = Wait (ms)(milliseconds to wait=u32 50) -> ()  [unwired: 1 out]
    n3274 = Or(x=w4199, y=w4200) -> (x .or. y?=w4201:bool)
    n3275 = case shown="True" w4201 {
      frame False {
      }
      frame True {
        n3276 = call <vilib>:"System Exec.vi"("run minimized? (F)"=TRUE, "error in (no error)"="error in (no error)", "command line"="powercfg.exe -change -monitor-timeout-ac 0") -> ("error out"=w4213:errorcluster)  [unwired: 5 in, 3 out]
        n3277 = call <vilib>:"System Exec.vi"("run minimized? (F)"=TRUE, "error in (no error)"=w4213, "command line"="powercfg.exe -change -disk-timeout-ac 0") -> ("error out"=w4212:errorcluster)  [unwired: 5 in, 3 out]
        n3278 = call <vilib>:"System Exec.vi"("run minimized? (F)"=TRUE, "error in (no error)"=w4212, "command line"="powercfg.exe -change -standby-timeout-ac 0") -> ("error out"=w4211:errorcluster)  [unwired: 5 in, 3 out]
        n3279 = call <vilib>:"System Exec.vi"("run minimized? (F)"=TRUE, "error in (no error)"=w4211, "command line"="powercfg.exe -change -hibernate-timeout-ac 0") -> ("error out"=w4210:errorcluster)  [unwired: 5 in, 3 out]
        n3280 = call <vilib>:"Simple Error Handler.vi"("error in (no error)"=w4210) -> ("error out"=w4216:errorcluster)  [unwired: 4 in, 4 out]
        n3281 = call <vilib>:"Clear Errors.vi"("error in (no error)"=w4216) -> ("error out"=→"error out":errorcluster)  [unwired: 5 in, 1 out]
      }
    }
  }
  n3282 = Compound Arithmetic op=OR(w59, w48, w56) -> (w58:bool)
  n3283 = flat-sequence {
    tunnel: w58 -> [_]
    tunnel: [w4218] -> w30
    tunnel: w30 -> [_]
    frame #0 {
      n3284 = call "CLOSE CONNECTION.vi"() -> ("error out"=w4218:errorcluster)  [unwired: 11 in]
    }
    frame #1 {
      n3285 = Quit LabVIEW(quit? (T)=TRUE) -> ()
      n3286 = local write "Quit"(FALSE ("EXIT")) -> ()
    }
  }
  n3287 = property on="Heater Button" class="Bool (strict)"("Visible"=TRUE) -> ()  [unwired: 2 in, 2 out]
  n3288 = while {
    tunnel: [w4225] -> _
    i -> [w4225]
    stop <- w4221 stop-if-true
    # "Langauage selection"
    n3289 = Equal?(x="Lan flag", y=22.0) -> ()  [unwired: 1 out]
    n3290 = disable-structure shown="Disabled" {
      frame Disabled {
        n3291 = stacked-sequence {
          frame #0 {
            n3292 = case shown="\"Russian\"" "Language Selection" {
              tunnel: [0 1] -> w4227
              frame "English", Default {
              }
              frame "Russian" {
              }
            }
            n3293 = for {
              N: 130 -> [_]
              tunnel: "Table" -> [w4236]
              tunnel: w4227 -> [w4235]
              i -> [w4234]
              n3294 = Index Array(array=w4236, index (row)=w4234, index (col)=w4235) -> (element=w4233:string)
              n3295 = case shown="1" w4234 {
                tunnel: w4233 -> [w4237 w4238 _ w4239 w4240 w4241 w4242 w4243 w4244 w4245 w4246 w4247 w4248 w4249 w4250 w4251 w4252 w4253 w4254 w4255 w4256 w4257 w4258 w4259 w4260 w4261 w4262 w4263 w4264 _ _ w4265 w4266 w4267 w4268 w4269 w4270 w4279 w4286 w4293 w4300 w4304 w4307 w4310 w4312 w4314 w4315 w4316 w4317 w4318 w4319 w4320 w4321 w4322 w4323 w4324 w4325 w4326 w4327 w4328 w4329 w4330 w4331 w4332 w4333 w4334 w4335 w4336 w4337 w4338 w4339 w4340 w4341 w4342 w4343 w4344 w4345 w4346 w4347 w4348 w4349 w4350 w4351 w4352 w4353 w4354 w4355 w4356 w4357 w4358 w4359 w4360 w4361 w4362 w4363 w4364 w4365 w4366 w4367 w4368 w4369 w4370 w4371 w4372 w4373 _ w4374 w4375 w4376 w4377 w4378 w4379 w4380 w4381 w4382 w4383 w4384 w4385 w4386 _ w4387 w4388 w4389 w4390 w4391 w4392 _]
                frame 0 {
                  n3296 = local write "S"(w4237) -> ()
                }
                frame 1 {
                  n3297 = local write "S 2"(w4238) -> ()
                }
                frame 2 {
                }
                frame 3 {
                  n3298 = local write "S 4"(w4239) -> ()
                }
                frame 4 {
                  n3299 = property on="FILE" class="Str"("Caption.Text"=w4240) -> ()  [unwired: 2 in, 2 out]
                }
                frame 5 {
                  n3300 = property on="Fuel Discription :" class="Str"("Caption.Text"=w4241) -> ()  [unwired: 2 in, 2 out]
                }
                frame 6 {
                  n3301 = property on="Remarks :" class="Str"("Caption.Text"=w4242) -> ()  [unwired: 2 in, 2 out]
                }
                frame 7 {
                  n3302 = property on="Save & Continue" class="Bool (strict)"("Boolean Text.Text"=w4243) -> ()  [unwired: 2 in, 2 out]
                }
                frame 8 {
                }
                frame 9 {
                  n3303 = property on="Set Hz" class="DigNum (strict)"("Caption.Text"=w4245) -> ()  [unwired: 2 in, 2 out]
                }
                frame 10 {
                }
                frame 11 {
                  n3304 = property on="NORMAL LOAD" class="DigNum (strict)"("Caption.Text"=w4247) -> ()  [unwired: 2 in, 2 out]
                }
                frame 12 {
                }
                frame 13 {
                  n3305 = property on="Set Temp" class="DigNum (strict)"("Caption.Text"=w4249) -> ()  [unwired: 2 in, 2 out]
                }
                frame 14 {
                  n3306 = local write "S 15"(w4250) -> ()
                }
                frame 15 {
                  n3307 = property on="Set Rh" class="DigNum (strict)"("Caption.Text"=w4251) -> ()  [unwired: 2 in, 2 out]
                }
                frame 16 {
                }
                frame 17 {
                  n3308 = local write "S 18"(w4253) -> ()
                }
                frame 18 {
                  "String 17" <- w4254
                }
                frame 19 {
                  n3309 = property on="test time" class="DigNum (strict)"("Caption.Text"=w4255) -> ()  [unwired: 2 in, 2 out]
                }
                frame 20 {
                  "String 18" <- w4256
                  "String 22" <- w4256
                }
                frame 21 {
                  n3310 = property on="Elapsed time" class="DigNum (strict)"("Caption.Text"=w4257) -> ()  [unwired: 2 in, 2 out]
                }
                frame 22 {
                  n3311 = property on="Samplingtime 2" class="DigNum (strict)"("Caption.Text"=w4258) -> ()  [unwired: 2 in, 2 out]
                }
                frame 23 {
                  "String 21" <- w4259
                }
                frame 24 {
                  n3312 = property on="Countdown" class="DigNum (strict)"("Caption.Text"=w4260) -> ()  [unwired: 2 in, 2 out]
                }
                frame 25 {
                  n3313 = property on="Countdown 2" class="DigNum (strict)"("Caption.Text"=w4261) -> ()  [unwired: 2 in, 2 out]
                }
                frame 26 {
                  n3314 = property on="Engage" class="Bool (strict)"("Boolean Text.Text"=w4262) -> ()  [unwired: 2 in, 2 out]
                }
                frame 27 {
                  n3315 = property on="Boolean  4" class="Bool (strict)"("Boolean Text.Text"=w4263) -> ()  [unwired: 2 in, 2 out]
                }
                frame 28 {
                  n3316 = property on="Test \nStatus" class="Bool (strict)"("Boolean Text.Text"=w4264) -> ()  [unwired: 2 in, 2 out]
                }
                frame 29 {
                }
                frame 30 {
                }
                frame 31 {
                }
                frame 32 {
                  n3317 = property on="RSTCOF" class="Bool"("Boolean Text.Text"=w4266) -> ()  [unwired: 2 in, 2 out]
                  n3318 = property on="RST FF" class="Bool"("Boolean Text.Text"=w4266) -> ()  [unwired: 2 in, 2 out]
                  n3319 = property on="RST TEMP" class="Bool"("Boolean Text.Text"=w4266) -> ()  [unwired: 2 in, 2 out]
                  n3320 = property on="RSTV1 3" class="Bool"("Boolean Text.Text"=w4266) -> ()  [unwired: 2 in, 2 out]
                  n3321 = property on="rstv2" class="Bool"("Boolean Text.Text"=w4266) -> ()  [unwired: 2 in, 2 out]
                  n3322 = property on="RSTV1 2" class="Bool"("Boolean Text.Text"=w4266) -> ()  [unwired: 2 in, 2 out]
                  n3323 = property on="RST CP" class="Bool"("Boolean Text.Text"=w4266) -> ()  [unwired: 2 in, 2 out]
                }
                frame 33 {
                  "S 61" <- w4267
                }
                frame 34 {
                  "String 23" <- w4268
                }
                frame 35 {
                  n3324 = property on="Rh Before" class="DigNum (strict)"("Caption.Text"=w4269) -> ()  [unwired: 2 in, 2 out]
                }
                frame 36 {
                  n3325 = Match Pattern(string=w4270, regular expression=",") -> (before substring=→"bs":string, after substring=→"as":string)  [unwired: 1 in, 2 out]
                  n3326 = property on="Rh After" class="DigNum (strict)"("Caption.Text"=w4270) -> ()  [unwired: 2 in, 2 out]
                }
                frame 37 {
                  n3327 = Match Pattern(string=w4279, regular expression=",") -> (before substring=w4278:string, after substring=w4277:string)  [unwired: 1 in, 2 out]
                  "bs" <- w4278
                  "as" <- w4277
                  n3328 = Concatenate Strings(w4278, w4277) -> (w4274:string)
                  n3329 = property on="Humidity before test 2" class="DigNum (strict)"("Caption.Text"=w4274) -> ()  [unwired: 2 in, 2 out]
                  n3330 = Concatenate Strings(w4274, "=" ("string")) -> (w4275:string)
                  n3331 = local write "S 38"(w4275) -> ()
                }
                frame 38 {
                  n3332 = Match Pattern(string=w4286, regular expression=",") -> (before substring=w4285:string, after substring=w4284:string)  [unwired: 1 in, 2 out]
                  "bs" <- w4285
                  "as" <- w4284
                  n3333 = Concatenate Strings(w4285, w4284) -> (w4281:string)
                  n3334 = property on="Humidity after test 2" class="DigNum (strict)"("Caption.Text"=w4281) -> ()  [unwired: 2 in, 2 out]
                  n3335 = Concatenate Strings(w4281, "=" ("string")) -> (w4283:string)
                  n3336 = local write "S 39"(w4283) -> ()
                }
                frame 39 {
                  n3337 = Match Pattern(string=w4293, regular expression=",") -> (before substring=w4292:string, after substring=w4291:string)  [unwired: 1 in, 2 out]
                  "bs" <- w4292
                  "as" <- w4291
                  n3338 = Concatenate Strings(w4292, w4291) -> (w4288:string)
                  n3339 = property on="Temperature before test 2" class="DigNum (strict)"("Caption.Text"=w4288) -> ()  [unwired: 2 in, 2 out]
                  n3340 = Concatenate Strings(w4288, "=" ("string")) -> (→"String 34":string)
                }
                frame 40 {
                  n3341 = Match Pattern(string=w4300, regular expression=",") -> (before substring=w4299:string, after substring=w4298:string)  [unwired: 1 in, 2 out]
                  "bs" <- w4299
                  "as" <- w4298
                  n3342 = Concatenate Strings(w4299, w4298) -> (w4295:string)
                  n3343 = property on="Temperature after test 2" class="DigNum (strict)"("Caption.Text"=w4295) -> ()  [unwired: 2 in, 2 out]
                  n3344 = Concatenate Strings(w4295, "=" ("string")) -> (→"String 35":string)
                  n3345 = property on="Temperature after test" class="DigNum (strict)"("Caption.Text"=w4295) -> ()  [unwired: 2 in, 2 out]
                }
                frame 41 {
                  n3346 = property on="AVP 2" class="DigNum (strict)"("Caption.Text"=w4304) -> ()  [unwired: 2 in, 2 out]
                  n3347 = Concatenate Strings(w4304, "=" ("string")) -> (→"String 36":string)
                }
                frame 42 {
                  n3348 = property on="MWSD 2" class="DigNum (strict)"("Caption.Text"=w4307) -> ()  [unwired: 2 in, 2 out]
                  n3349 = Concatenate Strings(w4307, "=" ("string")) -> (→"String 37":string)
                }
                frame 43 {
                  n3350 = property on="HCF 2" class="DigNum (strict)"("Caption.Text"=w4310) -> ()  [unwired: 2 in, 2 out]
                  n3351 = Concatenate Strings(w4310, "=" ("string")) -> (→"String 38":string)
                }
                frame 44 {
                  n3352 = Concatenate Strings(w4312, "=" ("string")) -> (→"String 39":string)
                  n3353 = property on="WS1.4 2" class="DigNum (strict)"("Caption.Text"=w4312) -> ()  [unwired: 2 in, 2 out]
                }
                frame 45 {
                }
                frame 46 {
                  n3354 = local write "S 47"(w4315) -> ()
                }
                frame 47 {
                  n3355 = local write "S 48"(w4316) -> ()
                }
                frame 48 {
                  n3356 = local write "S 49"(w4317) -> ()
                }
                frame 49 {
                  n3357 = local write "S 50"(w4318) -> ()
                }
                frame 50 {
                  n3358 = local write "S 51"(w4319) -> ()
                }
                frame 51 {
                  n3359 = local write "S 52"(w4320) -> ()
                }
                frame 52 {
                  n3360 = local write "S 53"(w4321) -> ()
                }
                frame 53 {
                  n3361 = local write "S 54"(w4322) -> ()
                }
                frame 54 {
                  n3362 = local write "S 55"(w4323) -> ()
                }
                frame 55 {
                  n3363 = local write "S 56"(w4324) -> ()
                }
                frame 56 {
                  n3364 = local write "S 57"(w4325) -> ()
                }
                frame 57 {
                  n3365 = local write "S 58"(w4326) -> ()
                }
                frame 58 {
                  n3366 = local write "S 59"(w4327) -> ()
                }
                frame 59 {
                  n3367 = local write "S 60"(w4328) -> ()
                }
                frame 60 {
                  n3368 = local write "S 62"(w4329) -> ()
                }
                frame 61 {
                  n3369 = local write "S 63"(w4330) -> ()
                }
                frame 62 {
                  n3370 = local write "S 64"(w4331) -> ()
                }
                frame 63 {
                  n3371 = local write "S 65"(w4332) -> ()
                }
                frame 64 {
                  n3372 = local write "S 66"(w4333) -> ()
                }
                frame 65 {
                  n3373 = local write "S 67"(w4334) -> ()
                }
                frame 66 {
                  n3374 = local write "S 68"(w4335) -> ()
                }
                frame 67 {
                  n3375 = local write "S 69"(w4336) -> ()
                }
                frame 68 {
                  n3376 = local write "S 70"(w4337) -> ()
                }
                frame 69 {
                  n3377 = local write "S 71"(w4338) -> ()
                }
                frame 70 {
                  n3378 = local write "S 72"(w4339) -> ()
                }
                frame 71 {
                  n3379 = local write "S 73"(w4340) -> ()
                }
                frame 72 {
                  n3380 = local write "S 74"(w4341) -> ()
                }
                frame 73 {
                  n3381 = local write "S 75"(w4342) -> ()
                }
                frame 74 {
                  n3382 = local write "S 76"(w4343) -> ()
                }
                frame 75 {
                  n3383 = local write "S 77"(w4344) -> ()
                }
                frame 76 {
                  n3384 = local write "S 78"(w4345) -> ()
                }
                frame 77 {
                  n3385 = local write "S 79"(w4346) -> ()
                }
                frame 79 {
                  n3386 = property on="Sample Temperature ( °C )" class="XYGraph (strict)"("Y Scale.Name Label.Text"=w4347) -> ()  [unwired: 2 in, 2 out]
                }
                frame 80 {
                  n3387 = local write "S 81"(w4348) -> ()
                  n3388 = property on="Humidity ( %RH )" class="XYGraph (strict)"("Y Scale.Name Label.Text"=w4348) -> ()  [unwired: 2 in, 2 out]
                }
                frame 78 {
                  n3389 = property on="Air Temperature  ( °C )" class="XYGraph (strict)"("X Scale.Name Label.Text"=w4349) -> ()  [unwired: 2 in, 2 out]
                  n3390 = property on="Humidity ( %RH )" class="XYGraph (strict)"("X Scale.Name Label.Text"=w4349) -> ()  [unwired: 2 in, 2 out]
                  n3391 = property on="Sample Temperature ( °C )" class="XYGraph (strict)"("X Scale.Name Label.Text"=w4349) -> ()  [unwired: 2 in, 2 out]
                  n3392 = property on="Coefficient Of Friction" class="XYGraph (strict)"("X Scale.Name Label.Text"=w4349) -> ()  [unwired: 2 in, 2 out]
                }
                frame 81 {
                  n3393 = property on="Air Temperature  ( °C )" class="XYGraph (strict)"("Y Scale.Name Label.Text"=w4350) -> ()  [unwired: 2 in, 2 out]
                }
                frame 82 {
                  n3394 = local write "S 84"(w4351) -> ()
                }
                frame 83 {
                  n3395 = local write "S 85"(w4352) -> ()
                }
                frame 84 {
                  n3396 = local write "S 86"(w4353) -> ()
                }
                frame 85 {
                  n3397 = local write "S 87"(w4354) -> ()
                }
                frame 86 {
                  n3398 = local write "S 88"(w4355) -> ()
                }
                frame 87 {
                }
                frame 88 {
                  n3399 = local write "S 90"(w4357) -> ()
                }
                frame 89 {
                  n3400 = local write "S 91"(w4358) -> ()
                }
                frame 90 {
                  n3401 = local write "S 92"(w4359) -> ()
                }
                frame 91 {
                  n3402 = local write "S 93"(w4360) -> ()
                }
                frame 92 {
                  n3403 = local write "S 94"(w4361) -> ()
                }
                frame 93 {
                  n3404 = local write "S 95"(w4362) -> ()
